vi "findfile File List Object.vi"(9 "size (20)":i32=20, 10 "Action (Add)":T2, 11 "Path":path) -> (2 "large?":bool, 3 "Largest Files":T1[](array[typedef]))   [LabVIEW 2011]
uses:
  findfile enum Action.ctl
  findfile cluster File and Size.ctl
panel:
  in  "files":T1
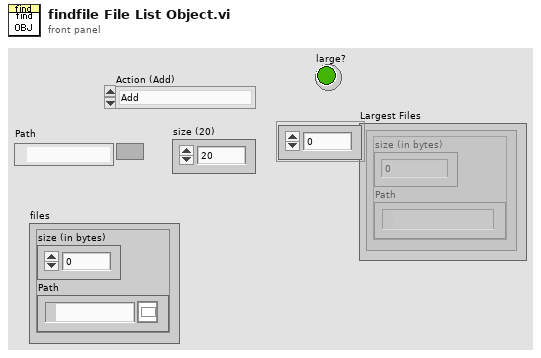
[diagram p1: front panel]
types:
  T1 = typedef "findfile cluster File and Size.ctl" = cluster{"size (in bytes)":i64, "Path":path}
  T2 = typedef "findfile enum Action.ctl" = enum16{"Add", "Read", "Reset"}
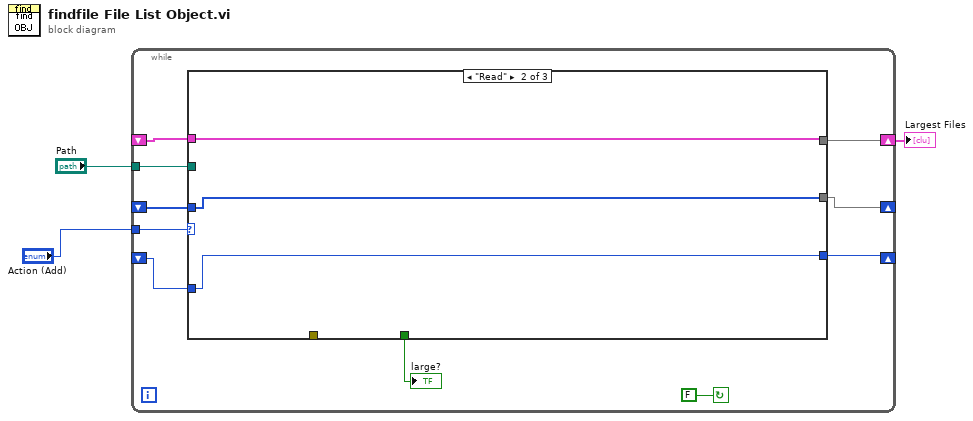
[diagram p0: block diagram]
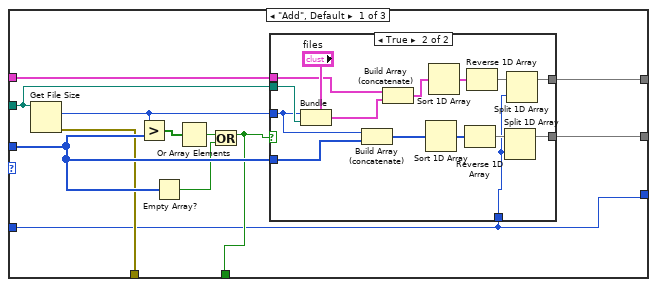
[diagram p2: hidden frame]
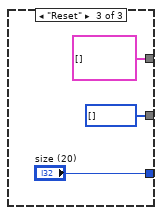
[diagram p4: hidden frame]
diagram:
  n1 = while {
    tunnel: "Path" -> [w12]
    tunnel: "Action (Add)" -> [w11]
    shift-right: [w10] -> _
    shift-left: _ -> [w9]
    shift-right: [w8] -> w1
    shift-left: _ -> [w7]
    shift-right: [w5] -> _
    shift-left: _ -> [w4]
    stop <- FALSE continue-if-true
    n2 = case shown="\"Read\"" w11 {
      tunnel: w12 -> [w21 _ _]
      tunnel: [w24 w44 i64[] []] -> w10
      tunnel: w9 -> [w18 w44 _]
      tunnel: [w20 w45 T1[] []] -> w8
      tunnel: w7 -> [w19 w45 _]
      tunnel: [w16 _ _] -> w6
      tunnel: [w15 _ _] -> _
      tunnel: [w14 w43 "size (20)"] -> w5
      tunnel: w4 -> [w14 w43 _]
      frame "Add", Default {
        n3 = Get File Size(file=w21) -> (size (in bytes)=w25:i64, 0:w15:errorcluster)  [unwired: 1 in, 1 out]
        n4 = Greater?(x=w25, y=w18) -> (0:w23:bool[])
        n5 = Empty Array?(array=w18) -> (empty?=w17:bool)
        n6 = Or Array Elements(Boolean array=w23) -> (logical OR=w22:bool)
        n7 = Or(x=w22, y=w17) -> (x .or. y?=w16:bool)
        n8 = case shown="True" w16 {
          tunnel: w25 -> [_ w39]
          tunnel: [w27 w29] -> w24
          tunnel: w21 -> [_ w41]
          tunnel: w18 -> [w27 w38]
          tunnel: [w26 w32] -> w20
          tunnel: w19 -> [w26 w35]
          tunnel: w14 -> [_ w28]
          frame False {
          }
          frame True {
            n9 = Bundle(cluster="files", "size (in bytes)"=w39, "Path"=w41) -> (w37:T1)
            n10 = Build Array (concatenate)(w39, w38) -> (w42:i64[])
            n11 = Build Array (concatenate)(w35, w37) -> (w36:T1[])
            n12 = Sort 1D Array(array=w42) -> (sorted array=w33:i64[])
            n13 = Sort 1D Array(array=w36) -> (sorted array=w34:T1[])
            n14 = Reverse 1D Array(array=w33) -> (reversed array=w30:i64[])
            n15 = Reverse 1D Array(array=w34) -> (reversed array=w31:T1[])
            n16 = Split 1D Array(array=w30, index=w28) -> (first subarray=w29:i64[])  [unwired: 1 out]
            n17 = Split 1D Array(array=w31, index=w28) -> (first subarray=w32:T1[])  [unwired: 1 out]
          }
        }
      }
      frame "Read" {
      }
      frame "Reset" {
      }
    }
    "large?" <- w6
  }
  "Largest Files" <- w1
